vi "DeltaT_2_Power1.vi"(8 "Longueur d'onde":dbl, 10 "Delta T":dbl) -> (2 "Power":dbl)   [LabVIEW 2022 SP3]
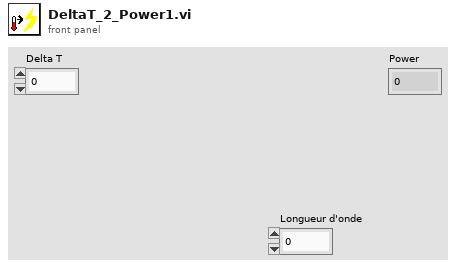
[diagram p1: front panel]
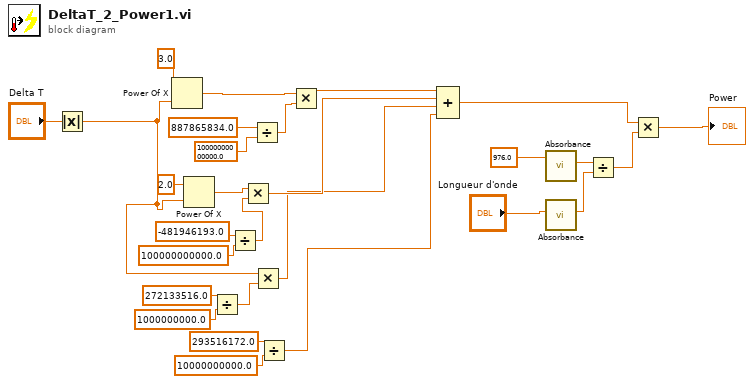
[diagram p0: block diagram]
diagram:
  n1 = Absolute Value(x="Delta T") -> (abs(x)=w9:dbl)
  n2 = Power Of X(1:w9, 2:3.0 ("y")) -> (0:w15:dbl)
  n3 = Power Of X(1:w9, 2:2.0 ("y")) -> (0:w23:dbl)
  n4 = Divide(x=272133516.0, y=1000000000.0) -> (x/y=w19:dbl)
  n5 = Divide(x=-481946193.0, y=100000000000.0) -> (x/y=w22:dbl)
  n6 = Multiply(x=w23, y=w22) -> (x*y=w12:dbl)
  n7 = Divide(x=887865834.0, y=10000000000000.0) -> (x/y=w14:dbl)
  n8 = Multiply(x=w9, y=w19) -> (x*y=w11:dbl)
  n9 = Divide(x=293516172.0, y=10000000000.0) -> (x/y=w10:dbl)
  n10 = Multiply(x=w15, y=w14) -> (x*y=w13:dbl)
  n11 = Compound Arithmetic op=ADD(w13, w12, w11, w10) -> (w3:dbl)
  n12 = call "Absorbance.vi"("Longueur d'onde"=976.0) -> ("absorbance"=w5:dbl)  [unwired: 10 in]
  n13 = call "Absorbance.vi"("Longueur d'onde"="Longueur d'onde") -> ("absorbance"=w4:dbl)  [unwired: 10 in]
  n14 = Divide(x=w5, y=w4) -> (x/y=w2:dbl)
  n15 = Multiply(x=w3, y=w2) -> (x*y=→"Power":dbl)
